vi "Write VI.vi"(8 "error in (no error)":errorcluster, 10 "Content in":T1, 11 "VI Path in":path) -> (0 "error out":errorcluster, 3 "VI Path out":path)   [LabVIEW 2021, in "VI-Hacker.lvlib"]
uses:
  VI-Hacker.lvlib
  TypeDefs/Content.ctl
  TypeDefs/Block.ctl
  <vilib>/Utility/error.llb/Error Cluster From Error Code.vi
  <vilib>/ErrorRing/Error Ring.xnode
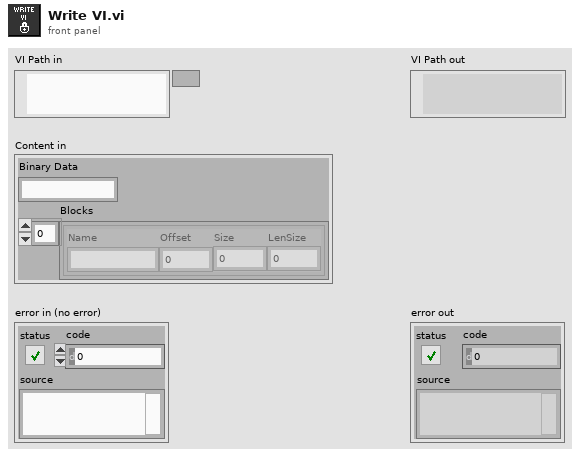
[diagram p1: front panel]
types:
  T1 = typedef "VI-Hacker.lvlib/Content.ctl" = cluster{"Binary Data":string, "Blocks":T2[]}
  T2 = typedef "VI-Hacker.lvlib/Block.ctl" = cluster{"Name":string, "Offset":i32, "Size":i32, "LenSize":i32}
  T3 = enum16{"open", "replace", "create", "open or create", "replace or create", "replace or create with confirmation"}
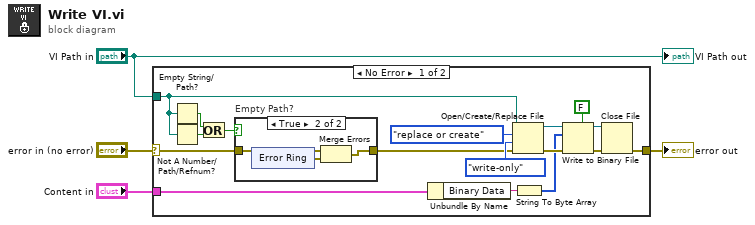
[diagram p0: block diagram]
diagram:
  n1 = case shown="No Error" "error in (no error)" {
    selector: "error in (no error)" -> [w12 w30]
    tunnel: "VI Path in" -> [w10 _]
    tunnel: [w9 w30] -> w3
    tunnel: "Content in" -> [w7 _]
    frame No Error {
      n2 = Empty String/Path?(string/path=w10) -> (empty?=w14:bool)
      n3 = Not A Number/Path/Refnum?(number/path/refnum=w10) -> (NaN/Path/Refnum?=w15:bool)
      n4 = Or(x=w14, y=w15) -> (x .or. y?=w13:bool)
      n5 = case "Empty Path?" shown="True" w13 {
        tunnel: w12 -> [w22 w25]
        tunnel: [w22 w24] -> w11
        frame False {
        }
        frame True {
          n6 = xnode "Error Ring"() -> ("error out"=w23:errorcluster)
          n7 = Merge Errors(w25, w23) -> (w24:errorcluster)
        }
      }
      n8 = Unbundle By Name(w7) -> ("Binary Data"=w6:string)
      n9 = Open/Create/Replace File(file path (use dialog)=w10, error in=w11, operation (0:open)=T3."replace or create", access (0:read/write)=enum16{"read/write", "read-only", "write-only"}."write-only") -> (refnum out=w16:refnum<file>, error out=w19:errorcluster)  [unwired: 3 out]
      n10 = String To Byte Array(string=w6) -> (unsigned byte array=w5:u8[])
      n11 = Write to Binary File(file (use dialog)=w16, data=w5, error in=w19, 5:FALSE ("prepend array or string size? (T)")) -> (refnum out=w18:refnum<file>, error out=w17:errorcluster)  [unwired: 2 in, 1 out]
      n12 = Close File(refnum=w18, error in=w17) -> (error out=w9:errorcluster)  [unwired: 1 out]
    }
    frame Error {
    }
  }
  "error out" <- w3
  "VI Path out" <- "VI Path in"
